vi "Title.vi"(4 "Properties":T1={"Text"={"Color"=2147483647, "Background Color"=2147483647, "Font Size (points)"=0, "Font Style"=enum."Automatic", "Rotation Angle"=nan}} {"Text"."Background Color" items=["Automatic"=2147483647, "Black"=0, "White"=16777215, "Red"=16711680, "Green"=2263842, "Blue"=255, "Cyan"=65535, "Magenta"=16711935, "Yellow"=16776960]; "Text"."Font Size (points)" items=["Automatic"=0, "XX-Small"=-1, "X-Small"=-2, "Small"=-3, "Medium"=-4, "Large"=-5, "X-Large"=-6, "XX-Large"=-7]; "Text"."Color" items=["Automatic"=2147483647, "Black"=0, "White"=16777215, "Red"=16711680, "Green"=2263842, "Blue"=255, "Cyan"=65535, "Magenta"=16711935, "Yellow"=16776960]}, 8 "error in (no error)":errorcluster, 10 "Title":string, 11 "Plot ID":T6 format="%x") -> (0 "error out":errorcluster, 3 "Plot ID out":T6 format="%x")   [LabVIEW 2013, in "Advanced Plotting Toolkit.lvlib"]
doc: "Set the plot title, which appears centered at the top of the axis box."
uses:
  Advanced Plotting Toolkit.lvlib
  typedefs/PlotID.ctl
  LabelProperties.ctl
  properties/Text.ctl
  typedefs/PlotColor.ctl
  properties/Text_FontSize.ctl
  properties/Text_FontStyle.ctl
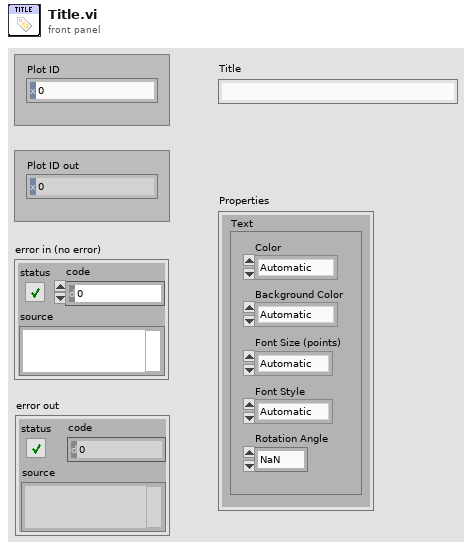
[diagram p1: front panel]
types:
  T1 = typedef "Advanced Plotting Toolkit.lvlib/LabelProperties.ctl" = cluster{"Text":T2}
  T2 = typedef "Advanced Plotting Toolkit.lvlib/Text.ctl" = cluster{"Color":T3, "Background Color":T3, "Font Size (points)":T4, "Font Style":T5, "Rotation Angle":dbl}
  T3 = typedef "Advanced Plotting Toolkit.lvlib/PlotColor.ctl" = u32
  T4 = typedef "Advanced Plotting Toolkit.lvlib/Text_FontSize.ctl" = i32
  T5 = typedef "Advanced Plotting Toolkit.lvlib/Text_FontStyle.ctl" = enum16{"Automatic", "Normal", "Italic", "Bold"}
  T6 = typedef "Advanced Plotting Toolkit.lvlib/PlotID.ctl" = i32
  T7 = enum16{"Plot Title", "X Axis Label", "Y Axis Label"}
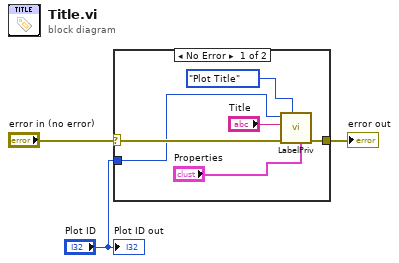
[diagram p0: block diagram]
diagram:
  n1 = case shown="No Error" "error in (no error)" {
    selector: "error in (no error)" -> [w7 w10]
    tunnel: "Plot ID" -> [w5 _]
    tunnel: [w6 w10] -> w1
    frame No Error {
      n2 = call "LabelPriv.vi"("Label Properties"="Properties", "Location"=T7."Plot Title", "error in (no error)"=w7, "Label"="Title", "Plot ID"=w5) -> ("error out"=w6:errorcluster)  [unwired: 6 in]
    }
    frame Error {
    }
  }
  "error out" <- w1
  "Plot ID out" <- "Plot ID"
